vi "Get SMU Buffer Size.vi"(0 "SMU":string, 5 "No. of steps":i32, 11 "error in (no error)":errorcluster) -> (4 "Required Buffer Size":i32, 6 "Maximum Buffer Size":i32, 10 "Insufficient Memory":bool, 15 "error out":errorcluster)   [LabVIEW 2020, in "LDO Load Transient_AWG.lvlib"]
uses:
  LDO Load Transient_AWG.lvlib
  ea803309-b67d-47c3-a957-add2e4a95a09.vi
  <userlib>/_Soliton/Measurement Suite/Reusables/InstrumentSessionAPIs/SessionManagerApiPath.vi
  <vilib>/Utility/sysdir.llb/Get System Directory.vi
  <vilib>/Utility/LVLibp/Get Exported File Path.vi
  <userlib>/_Soliton/Measurement Suite/Reusables/Errors/Error 6001.vi
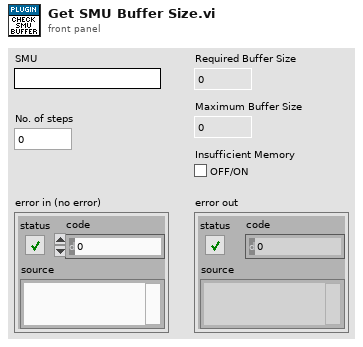
[diagram p1: front panel]
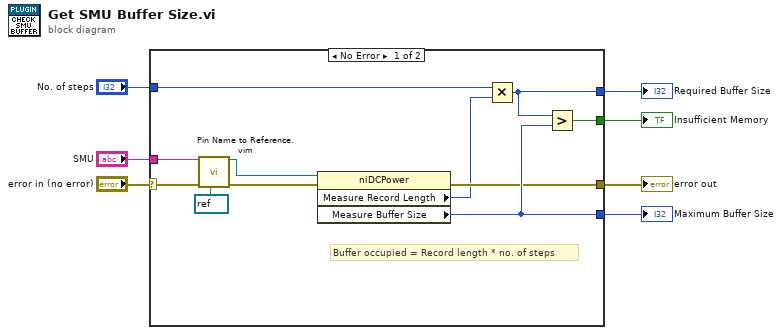
[diagram p0: block diagram]
diagram:
  n1 = case shown="No Error" "error in (no error)" {
    selector: "error in (no error)" -> [w11 w19]
    tunnel: [w18 _] -> w7
    tunnel: [w17 _] -> w6
    tunnel: [w16 _] -> w5
    tunnel: [w15 w19] -> w4
    tunnel: "No. of steps" -> [w14 _]
    tunnel: "SMU" -> [w8 _]
    frame No Error {
      # "Buffer occupied = Record length * no. of steps"
      n2 = call "Pin Name to Reference.vim"("Pin Name"=w8, "type"=refnum<k15> refnum ("instrument handle"), "error in (no error)"=w11) -> ("Reference"=w9:refnum<k15>, "error out"=w10:errorcluster)  [unwired: 7 in, 4 out]
      n3 = property class="niDCPower"(reference=w9, error in=w10) -> (error out=w15:errorcluster, "Measure Record Length"=w13:i32, "Measure Buffer Size"=w17:i32)  [unwired: 1 out]
      n4 = Multiply(x=w14, y=w13) -> (x*y=w16:i32)
      n5 = Greater?(x=w16, y=w17) -> (0:w18:bool)
    }
    frame Error {
    }
  }
  "Insufficient Memory" <- w7
  "Maximum Buffer Size" <- w6
  "Required Buffer Size" <- w5
  "error out" <- w4
